vi "Drop.vi"(11 "Response Core in":refnum<class "Response Core.lvclass">) -> ()   [LabVIEW 2020, in "Publisher.lvlib" / "Response Core.lvclass"]
doc: "Drop the Response Core.\n\nThe default implementation does nothing."
uses:
  Response Core.lvclass
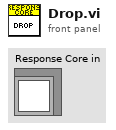
[diagram p1: front panel]
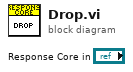
[diagram p0: block diagram]
diagram:
